vi "getViReference.vi"(6 "vi reference in":refnum<vi>, 8 "error in (no error)":errorcluster, 9 "Path":path, 10 "vi":string, 11 "ProgrammaticInitialization in":refnum<class "ProgrammaticInitialization.lvclass">) -> (0 "error out":errorcluster, 2 "vi reference in 2":variant, 3 "ProgrammaticInitialization out":refnum<class "ProgrammaticInitialization.lvclass">)   [LabVIEW 2016, in "ProgrammaticInitialization.lvclass"]
uses:
  ProgrammaticInitialization.lvclass
  ProgrammaticInitialization.lvclass/ProgrammaticInitialization.ctl
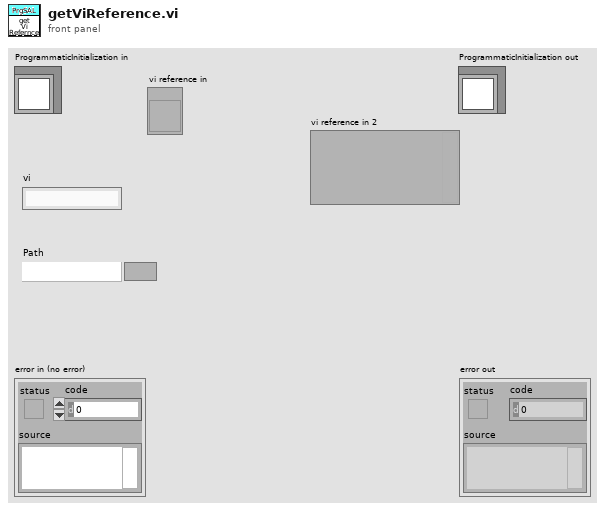
[diagram p1: front panel]
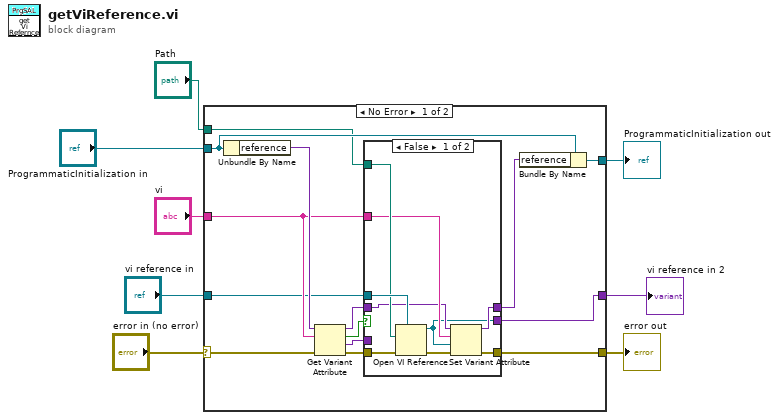
[diagram p0: block diagram]
diagram:
  n1 = case shown="No Error" "error in (no error)" {
    selector: "error in (no error)" -> [w19 w37]
    tunnel: [w18 w37] -> w7
    tunnel: [w14 w36] -> w5
    tunnel: "ProgrammaticInitialization in" -> [w13 w36]
    tunnel: "vi" -> [w11 _]
    tunnel: "vi reference in" -> [w9 w35]
    tunnel: "Path" -> [w12 _]
    tunnel: [w10 w35] -> w1
    frame No Error {
      n2 = Unbundle By Name(w13) -> ("reference"=w17:variant)
      n3 = Get Variant Attribute(Variant=w17, name=w11, error in=w19) -> (duplicate Variant=w16:variant, found=w22:bool, value=w20:variant, error out=w21:errorcluster)  [unwired: 1 in]
      n4 = case shown="False" w22 {
        tunnel: w21 -> [w29 w34]
        tunnel: w20 -> [_ w32]
        tunnel: [w31 w34] -> w18
        tunnel: w16 -> [w24 w33]
        tunnel: [w30 w33] -> w15
        tunnel: w9 -> [w27 _]
        tunnel: w12 -> [w26 _]
        tunnel: w11 -> [w25 _]
        tunnel: [w23 w32] -> w10
        frame False {
          n5 = Open VI Reference(type specifier VI Refnum (for type only)=w27, vi path=w26, error in (no error)=w29) -> (vi reference=w23:refnum<vi>, error out=w28:errorcluster)  [unwired: 3 in]
          n6 = Set Variant Attribute(Variant=w24, name=w25, value=w23, error in=w28) -> (Variant out=w30:variant, error out=w31:errorcluster)  [unwired: 1 out]
        }
        frame True {
        }
      }
      n7 = Bundle By Name(cluster=w13, "reference"=w15) -> (w14:refnum<class "ProgrammaticInitialization.lvclass">)
    }
    frame Error {
    }
  }
  "error out" <- w7
  "ProgrammaticInitialization out" <- w5
  "vi reference in 2" <- w1
